vi "LEDExecute.vi"() -> ()   [LabVIEW 2023]
uses:
  <vilib>/Rock Robotics/WPI/DriverStation/WPI_DriverStationAllianceInfo.ctl
  TheBox/BoxNoteState.ctl
  Human/HumanGlobal.vi
  <vilib>/Rock Robotics/WPI/ThirdParty/PhotonVisionLib/PhotonVisionLib.lvlib
panel:
  out "Numeric":i32
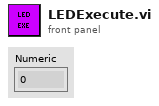
[diagram p1: front panel]
types:
  T1 = typedef "BoxNoteState.ctl" = enum16{"note in shooter wheels", "misaligned note", "no note", "have note"}
  T2 = typedef "WPI_DriverStationAllianceInfo.ctl" = enum16{"Red", "Blue", "Invalid"}
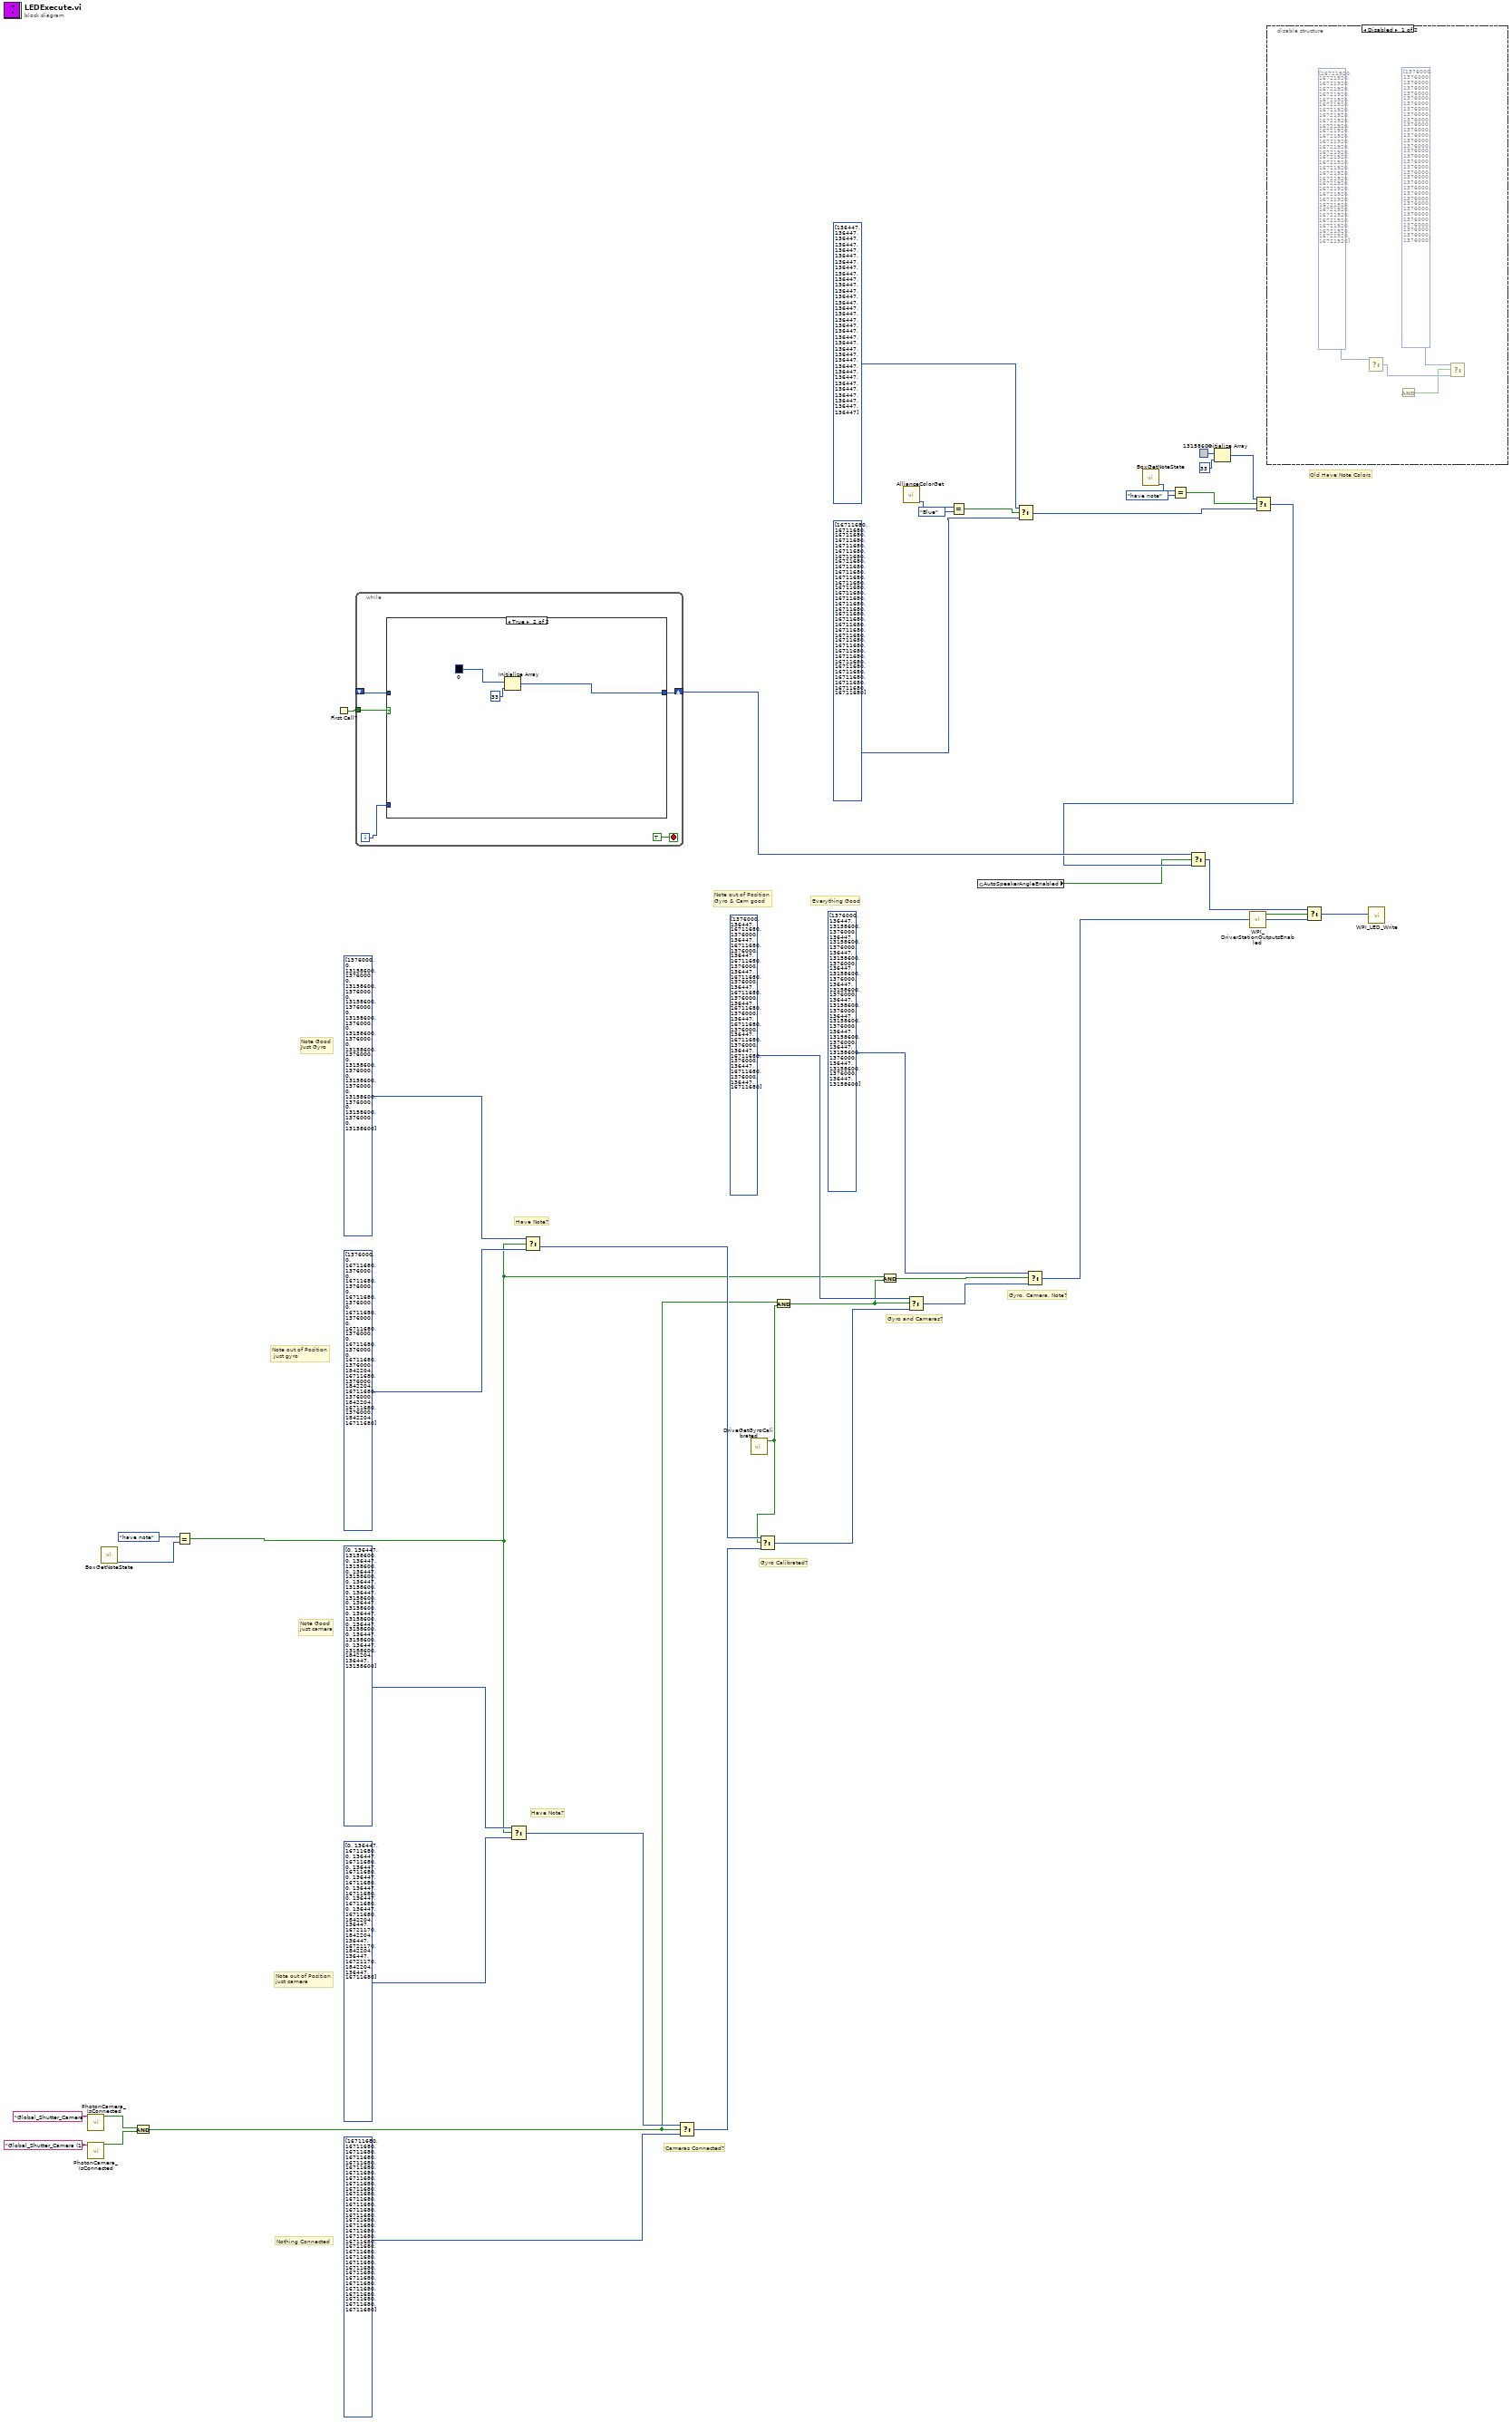
[diagram p0: block diagram]
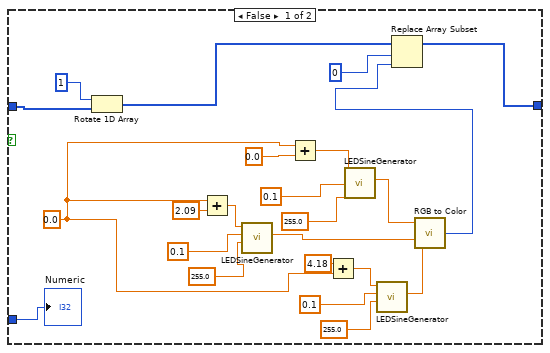
[diagram p2: hidden frame]
diagram:
  # "Old Have Note Colors"
  # "Gyro, Camera, Note?"
  # "Gyro and Cameras?"
  # "Gyro Calibrated?"
  # "Cameras Connected?"
  # "Have Note?"
  # "Have Note?"
  # "Note Good\njust camera"
  # "Note Good\nJust Gyro"
  # "Note out of Position\n just gyro"
  # "Note out of Position\njust camera"
  # "Everything Good"
  # "Note out of Position\nGyro & Cam good"
  # "Nothing Connected"
  n1 = call <vilib>:"PhotonCamera_IsConnected.vi"("CameraName"="Global_Shutter_Camera") -> ("IsConnected"=w24:bool)  [unwired: 9 in, 1 out]
  n2 = call <vilib>:"PhotonCamera_IsConnected.vi"("CameraName"="Global_Shutter_Camera (1)") -> ("IsConnected"=w23:bool)  [unwired: 9 in, 1 out]
  n3 = call "BoxGetNoteState.vi"() -> ("Box Note State"=w14:T1)  [unwired: 11 in]
  n4 = And(x=w24, y=w23) -> (x .and. y?=w27:bool)
  n5 = Equal?(x=BoxNoteState."have note" ("y"), y=w14) -> (x = y?=w1:bool)
  n6 = First Call?() -> (First Call?: T/F=w10:bool)
  n7 = while {
    tunnel: w10 -> [w47]
    shift-right: [w46] -> w8
    shift-left: _ -> [w45]
    i -> [w44]
    stop <- TRUE stop-if-true
    n8 = case shown="True" w47 {
      tunnel: [w62 w72] -> w46
      tunnel: w45 -> [w71 _]
      tunnel: w44 -> [w61 _]
      frame False {
        w65 = 0.0
        n9 = Rotate 1D Array(1:w71, 2:1 ("n")) -> (0:w69:u32[])
        n10 = Add(x=w65, y=2.09 ("Speed")) -> (x+y=w56:dbl)
        n11 = call "LEDSineGenerator.vi"("Amplitude"=255.0, "Speed"=0.1 ("Delay"), "Delay"=w56) -> ("Output"=w53:dbl)  [unwired: 8 in]
        n12 = Add(x=w65, y=0.0 ("Speed")) -> (x+y=w60:dbl)
        n13 = Add(x=4.18 ("Speed"), y=w65) -> (x+y=w52:dbl)
        n14 = call "LEDSineGenerator.vi"("Amplitude"=255.0, "Speed"=0.1 ("Delay"), "Delay"=w60) -> ("Output"=w57:dbl)  [unwired: 8 in]
        n15 = call "LEDSineGenerator.vi"("Amplitude"=255.0, "Speed"=0.1 ("Delay"), "Delay"=w52) -> ("Output"=w49:dbl)  [unwired: 8 in]
        n16 = call <vilib>:"RGB to Color.vi"("B"=w49, "G"=w53, "R"=w57) -> ("Color"=w64:u32)
        n17 = Replace Array Subset(array=w69, new element=w64, index=0) -> (w62:u32[])
        "Numeric" <- w61
      }
      frame True {
        n18 = Initialize Array(u32 0 ("Color Box 3"), 33 ("dimension size")) -> (w72:u32[])
      }
    }
  }
  n19 = Select(t=u32[] [0, 136447, 13158600, 0, 136447, 13158600, 0, 136447, 13158600, 0, 136447, 13158600, 0, 136447, 13158600, 0, 136447, 13158600, 0, 136447, 13158600, 0, 136447, 13158600, 0, 136447, 13158600, 0, 136447, 13158600, 1842204, 136447, 13158600] ("Color Array"), s=w1, f=u32[] [0, 136447, 16711680, 0, 136447, 16711680, 0, 136447, 16711680, 0, 136447, 16711680, 0, 136447, 16711680, 0, 136447, 16711680, 0, 136447, 16711680, 1842204, 136447, 16721170, 1842204, 136447, 16721170, 1842204, 136447, 16721170, 1842204, 136447, 16711680] ("Color Array")) -> (s? t:f=w36:u32[])
  n20 = Select(t=u32[] [1376000, 0, 13158600, 1376000, 0, 13158600, 1376000, 0, 13158600, 1376000, 0, 13158600, 1376000, 0, 13158600, 1376000, 0, 13158600, 1376000, 0, 13158600, 1376000, 0, 13158600, 1376000, 0, 13158600, 1376000, 0, 13158600, 1376000, 0, 13158600] ("Color Array"), s=w1, f=u32[] [1376000, 0, 16711680, 1376000, 0, 16711680, 1376000, 0, 16711680, 1376000, 0, 16711680, 1376000, 0, 16711680, 1376000, 0, 16711680, 1376000, 0, 16711680, 1376000, 1842204, 16711680, 1376000, 1842204, 16711680, 1376000, 1842204, 16711680, 1376000, 1842204, 16711680] ("Color Array")) -> (s? t:f=w38:u32[])
  n21 = Select(t=w36, s=w27, f=u32[] [16711680, 16711680, 16711680, 16711680, 16711680, 16711680, 16711680, 16711680, 16711680, 16711680, 16711680, 16711680, 16711680, 16711680, 16711680, 16711680, 16711680, 16711680, 16711680, 16711680, 16711680, 16711680, 16711680, 16711680, 16711680, 16711680, 16711680, 16711680, 16711680, 16711680, 16711680, 16711680, 16711680] ("Color Array")) -> (s? t:f=w43:u32[])
  n22 = call "DriveGetGyroCalibrated.vi"() -> ("GryoCalibrated"=w22:bool)  [unwired: 11 in]
  n23 = Select(t=w38, s=w22, f=w43) -> (s? t:f=w41:u32[])
  n24 = And(x=w27, y=w22) -> (x .and. y?=w29:bool)
  n25 = And(x=w1, y=w29) -> (x .and. y?=w28:bool)
  n26 = call "AllianceColorGet.vi"() -> ("AllianceColor"=w21:T2)  [unwired: 11 in]
  n27 = Select(t=u32[] [1376000, 136447, 16711680, 1376000, 136447, 16711680, 1376000, 136447, 16711680, 1376000, 136447, 16711680, 1376000, 136447, 16711680, 1376000, 136447, 16711680, 1376000, 136447, 16711680, 1376000, 136447, 16711680, 1376000, 136447, 16711680, 1376000, 136447, 16711680, 1376000, 136447, 16711680] ("Color Array"), s=w29, f=w41) -> (s? t:f=w33:u32[])
  n28 = Equal?(x=w21, y=WPI_DriverStationAllianceInfo."Blue") -> (x = y?=w15:bool)
  n29 = global read "HumanGlobal.vi" "AutoSpeakerAngleEnabled"() -> (w2:bool)
  n30 = Select(t=u32[] [136447, 136447, 136447, 136447, 136447, 136447, 136447, 136447, 136447, 136447, 136447, 136447, 136447, 136447, 136447, 136447, 136447, 136447, 136447, 136447, 136447, 136447, 136447, 136447, 136447, 136447, 136447, 136447, 136447, 136447, 136447, 136447, 136447] ("Color Array"), s=w15, f=u32[] [16711680, 16711680, 16711680, 16711680, 16711680, 16711680, 16711680, 16711680, 16711680, 16711680, 16711680, 16711680, 16711680, 16711680, 16711680, 16711680, 16711680, 16711680, 16711680, 16711680, 16711680, 16711680, 16711680, 16711680, 16711680, 16711680, 16711680, 16711680, 16711680, 16711680, 16711680, 16711680, 16711680] ("Color Array")) -> (s? t:f=w9:u32[])
  n31 = Select(t=u32[] [1376000, 136447, 13158600, 1376000, 136447, 13158600, 1376000, 136447, 13158600, 1376000, 136447, 13158600, 1376000, 136447, 13158600, 1376000, 136447, 13158600, 1376000, 136447, 13158600, 1376000, 136447, 13158600, 1376000, 136447, 13158600, 1376000, 136447, 13158600, 1376000, 136447, 13158600] ("Color Array"), s=w28, f=w33) -> (s? t:f=w32:u32[])
  n32 = call "BoxGetNoteState.vi"() -> ("Box Note State"=w17:T1)  [unwired: 11 in]
  n33 = Equal?(x=w17, y=BoxNoteState."have note") -> (x = y?=w12:bool)
  n34 = Initialize Array(u32 13158600 ("Color Box 3"), 33 ("dimension size")) -> (w3:u32[])
  n35 = call <vilib>:"WPI_DriverStationOutputsEnabled.vi"() -> ("OutputsEnabled?"=w40:bool)  [unwired: 10 in, 1 out]
  n36 = Select(t=w3, s=w12, f=w9) -> (s? t:f=w7:u32[])
  n37 = Select(t=w8, s=w2, f=w7) -> (s? t:f=w6:u32[])
  n38 = disable-structure shown="Disabled" {
    frame Disabled {
      n39 = Select(t=u32[] [16721920, 16721920, 16721920, 16721920, 16721920, 16721920, 16721920, 16721920, 16721920, 16721920, 16721920, 16721920, 16721920, 16721920, 16721920, 16721920, 16721920, 16721920, 16721920, 16721920, 16721920, 16721920, 16721920, 16721920, 16721920, 16721920, 16721920, 16721920, 16721920, 16721920, 16721920, 16721920, 16721920] ("Color Array")) -> (s? t:f=w75:u32[])  [unwired: 2 in]
      n40 = And() -> (x .and. y?=w76:bool)  [unwired: 2 in]
      n41 = Select(t=u32[] [1376000, 1376000, 1376000, 1376000, 1376000, 1376000, 1376000, 1376000, 1376000, 1376000, 1376000, 1376000, 1376000, 1376000, 1376000, 1376000, 1376000, 1376000, 1376000, 1376000, 1376000, 1376000, 1376000, 1376000, 1376000, 1376000, 1376000, 1376000, 1376000, 1376000, 1376000, 1376000, 1376000] ("Color Array"), s=w76, f=w75) -> ()  [unwired: 1 out]
    }
    frame Enabled {
    }
  }
  n42 = Select(t=w6, s=w40, f=w32) -> (s? t:f=w11:u32[])
  n43 = call <vilib>:"WPI_LED_Write.vi"("Color Array"=w11) -> ()  [unwired: 10 in, 1 out]
